vi "Configuration Keys.vi"(8 "error in":errorcluster, 11 "Instruments in":refnum<class "Instruments.lvclass">) -> (0 "error out":errorcluster, 2 "Required Keys":string[](array[string]), 3 "Instruments out":refnum<class "Instruments.lvclass">)   [LabVIEW 2023, in "Instruments.lvlib" / "Instruments.lvclass"]
doc: "Configuration Keys is a dynamic dispatch VI that reads a full inheritance chain's required key list.\n\nThis means each instrument must override this vi, and call the parent method . The end result is a comprehensive list of required keys that must be present in an instrument's config.ini file to correctly function."
uses:
  Library/Instruments.lvclass
  Custom Controls/ConfigurationKeys.ctl
  builds/Tools/Config.lvlibp/Config.lvclass
panel:
  in  "Configuration Keys":T1
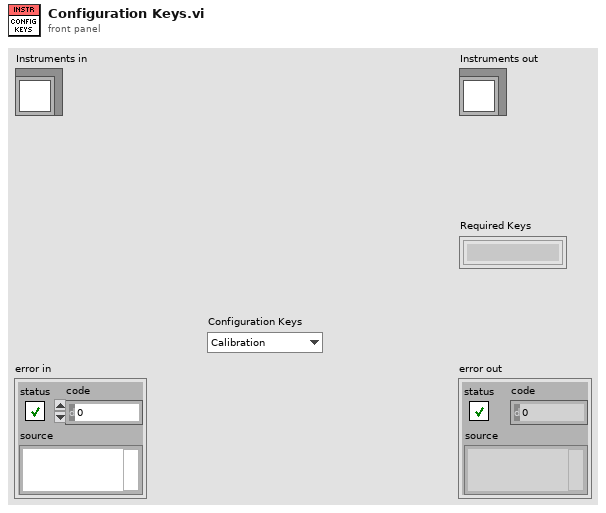
[diagram p1: front panel]
types:
  T1 = typedef "Instruments.lvlib/Instruments.lvclass/ConfigurationKeys.ctl" = enum16{"Calibration", "Resource", "Poll(ms)", "Panel", "Simulated", "Enabled"}
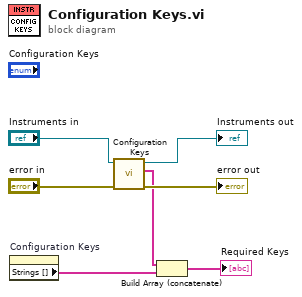
[diagram p0: block diagram]
diagram:
  n1 = property on="Configuration Keys" class="Enum (strict)"() -> ("Strings []"=w1:string[])  [unwired: 2 in, 2 out]
  n2 = call-parent "Configuration Keys.vi"("error in (no error)"="error in", "Config in"="Instruments in") -> ("error out"=→"error out":errorcluster, "Required Keys"=w3:string[], "Config out"=→"Instruments out":refnum<class "Instruments.lvclass">)  [unwired: 7 in]
  n3 = Build Array (concatenate)(w3, w1) -> (→"Required Keys":string[])
